vi "FA_Create_New_Teams.vi"(8 "error in (no error)":errorcluster, 11 "XML String":string) -> (0 "error out":errorcluster)   [LabVIEW 2013, in "FA_FIRST.lvlib"]
uses:
  FA_FIRST.lvlib
  FIRST Client/source/VI Source/FC_Team Attributes.ctl
  Backend/source/VI Source/FRCts20_Backend_API/FRCts20_Backend_API_Command_TeamRoot.ctl
  Backend/source/VI Source/FRCts20_Backend_API/FRCts20_Backend_API_TeamRoot.ctl
  Backend/source/VI Source/FRCts20_Backend_API/FRCts20_Backend_API_SW.ctl
  Backend/source/VI Source/FRCts20_Backend_API/FRCts20_Backend_API_TeamRoot.vi
  Backend/source/VI Source/FRCts20_Backend_API/FRCts20_Backend_API.lvlib
  FIRST Client/source/VI Source/FC_FIRST Client.lvlib
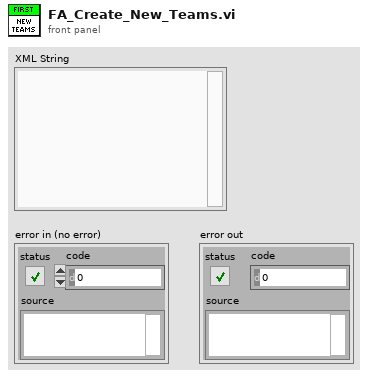
[diagram p1: front panel]
types:
  T1 = typedef "FRCts20_Backend_API.lvlib/FRCts20_Backend_API_TeamRoot.ctl" = cluster{"Teams":cluster{"Team Index":u32, "Team Number":u32, "Team ID":u32, "Team Name":string, "Short Team Name":string, "Nick Name":string, "Robot Name":string, "City":string, "State":string, "Country":string, "Rookie Year":u32, "SWType":T2, "CAN":bool, "Vision":bool, "Kinect":bool, "Tags":string, "Avatar":string, "Events":cluster{"EventIndex":u32, "EventName":string, "IsLive":bool}[]}[], "APIReturn":string}
  T2 = typedef "FRCts20_Backend_API.lvlib/FRCts20_Backend_API_SW.ctl" = string
  T3 = typedef "FRCts20_Backend_API.lvlib/FRCts20_Backend_API_Command_TeamRoot.ctl" = string
  T4 = typedef "FC_FIRST Client.lvlib/FC_Team Attributes.ctl" = cluster{"Team ID":string, "Team #":string, "Team Name":string, "Short Team Name":string, "City":string, "State":string, "Country":string, "Nickname":string, "Rookie Year":string, "Robot Name":string}
  T5 = cluster{"Team Index":u32, "Team Number":u32, "Team ID":u32, "Team Name":string, "Short Team Name":string, "Nick Name":string, "Robot Name":string, "City":string, "State":string, "Country":string, "Rookie Year":u32, "SWType":T2, "CAN":bool, "Vision":bool, "Kinect":bool, "Tags":string, "Avatar":string, "Events":cluster{"EventIndex":u32, "EventName":string, "IsLive":bool}[]}[]
  T6 = cluster{"Team Index":u32, "Team Number":u32, "Team ID":u32, "Team Name":string, "Short Team Name":string, "Nick Name":string, "Robot Name":string, "City":string, "State":string, "Country":string, "Rookie Year":u32, "SWType":T2, "CAN":bool, "Vision":bool, "Kinect":bool, "Tags":string, "Avatar":string, "Events":cluster{"EventIndex":u32, "EventName":string, "IsLive":bool}[]}
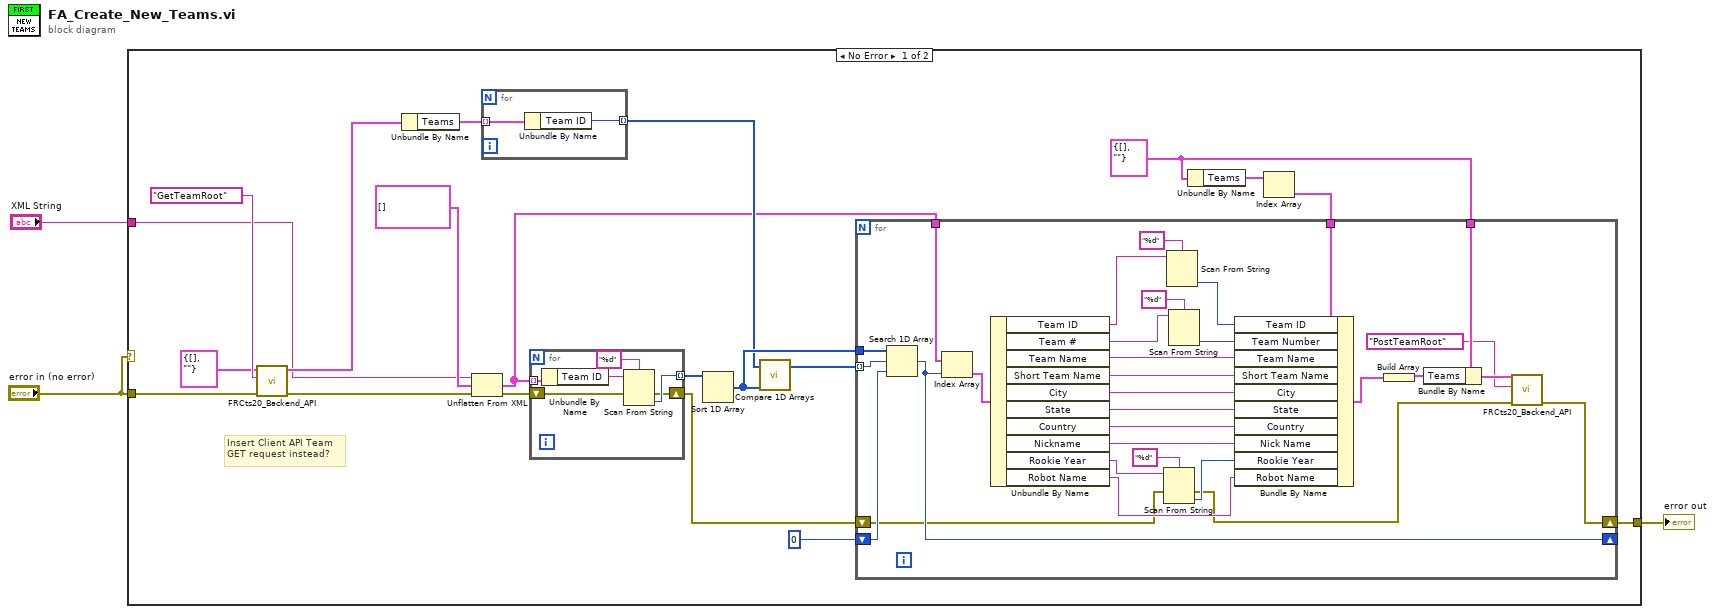
[diagram p0: block diagram]
diagram:
  n1 = case shown="No Error" "error in (no error)" {
    tunnel: [w23 _] -> w3
    tunnel: "error in (no error)" -> [w19 _]
    tunnel: "XML String" -> [w8 _]
    frame No Error {
      w5 = T1 {"Teams"=[], "APIReturn"=""} ("Team In")
      # "Insert Client API Team\nGET request instead?"
      n2 = call-poly "FRCts20_Backend_API.vi"("error in (no error)"=w19, "Command"=T3 "GetTeamRoot", "Team In"=T1 {"Teams"=[], "APIReturn"=""}) -> ("error out"=w22:errorcluster, "Team Out"=w21:T1)  [unwired: 6 in, 1 out]
      n3 = Unbundle By Name(w21) -> ("Teams"=w20:T5)
      n4 = Unflatten From XML(xml string=w8, type=T4[] [], error in (no error)=w22) -> (value=w6:T4[], error out=w15:errorcluster)
      n5 = for {
        tunnel: [w62] -> w11 mode=indexing
        tunnel: w20 -> [w61] mode=indexing
        n6 = Unbundle By Name(w61) -> ("Team ID"=w62:u32)
      }
      n7 = for {
        tunnel: w6 -> [w60] mode=indexing
        tunnel: [w57] -> w10 mode=indexing
        shift-right: [w55] -> w16
        shift-left: w15 -> [w56]
        n8 = Unbundle By Name(w60) -> ("Team ID"=w59:string)
        n9 = Scan From String(format string="%d", input string=w59, error in=w56) -> (error out=w55:errorcluster, output 1=w57:i32)  [unwired: 2 in, 2 out]
      }
      n10 = Sort 1D Array(array=w10) -> (sorted array=w12:i32[])
      n11 = call "Compare 1D Arrays.vi"("New Array"=w12, "Old Array"=w11) -> ("Added"=w9:i32[])  [unwired: 1 out]
      n12 = Unbundle By Name(w5) -> ("Teams"=w4:T5)
      n13 = Index Array(array=w4) -> (element=w17:T6)  [unwired: 1 in]
      n14 = for {
        shift-right: [w53] -> _
        shift-left: 0 ("index of element") -> [w54]
        tunnel: w9 -> [w30] mode=indexing
        tunnel: w12 -> [w52]
        tunnel: w6 -> [w51]
        shift-right: [w41] -> w23
        shift-left: w16 -> [w32]
        tunnel: w17 -> [w47]
        tunnel: w5 -> [w36]
        n15 = Search 1D Array(1D array=w52, element=w30, start index (0)=w54) -> (index of element=w53:i32)
        n16 = Index Array(array=w51, index=w53) -> (element=w50:T4)
        n17 = Unbundle By Name(w50) -> ("Team ID"=w25:string, "Team #"=w28:string, "Team Name"=w49:string, "Short Team Name"=w48:string, "City"=w46:string, "State"=w45:string, "Country"=w44:string, "Nickname"=w43:string, "Rookie Year"=w39:string, "Robot Name"=w42:string)
        n18 = Scan From String(format string="%d", input string=w39, error in=w32) -> (error out=w31:errorcluster, output 1=w38:i32)  [unwired: 2 in, 2 out]
        n19 = Scan From String(format string="%d", input string=w25) -> (output 1=w24:i32)  [unwired: 3 in, 3 out]
        n20 = Scan From String(format string="%d", input string=w28) -> (output 1=w27:i32)  [unwired: 3 in, 3 out]
        n21 = Bundle By Name(cluster=w47, "Team ID"=w24, "Team Number"=w27, "Team Name"=w49, "Short Team Name"=w48, "City"=w46, "State"=w45, "Country"=w44, "Nick Name"=w43, "Rookie Year"=w38, "Robot Name"=w42) -> (w37:T6)
        n22 = Build Array(w37) -> (w35:T5)
        n23 = Bundle By Name(cluster=w36, "Teams"=w35) -> (w34:T1)
        n24 = call-poly "FRCts20_Backend_API.vi"("error in (no error)"=w31, "Command"=T3 "PostTeamRoot", "Team In"=w34) -> ("error out"=w41:errorcluster)  [unwired: 6 in, 2 out]
      }
    }
    frame Error {
    }
  }
  "error out" <- w3
